vi "Material-Application-Constants.vi"() -> ()   [LabVIEW 2013]
panel:
  in  "Plugin Filename Pattern":string="Plugin-???-*.vi"
  in  "License Server Sandbox Request URI":string="https://apps.wirebirdlabs.com/license/deploy/sandbox"
  in  "License Server Registration URI":string="https://apps.wirebirdlabs.com/license/deploy/register"
  in  "Deploy Update Service Manifest URI":string="http://deploy.wirebirdlabs.com/OfficialReleases.manifest"
  out "Color.BG.Normal":u32(colorbox)=16777215
  out "Color.Selection":u32(colorbox)=16777224
  out "Color.BG.Fail":u32(colorbox)=16763594
  out "Color.BG.Success":u32(colorbox)=15204311
  out "Color.Text.Normal":u32(colorbox)=4276545
  out "Color.Text.Fail":u32(colorbox)=12517376
  out "Color.Text.Success":u32(colorbox)=3176192
  # "Colors"
  # "Endpoints"
  # "Plugin Constants"
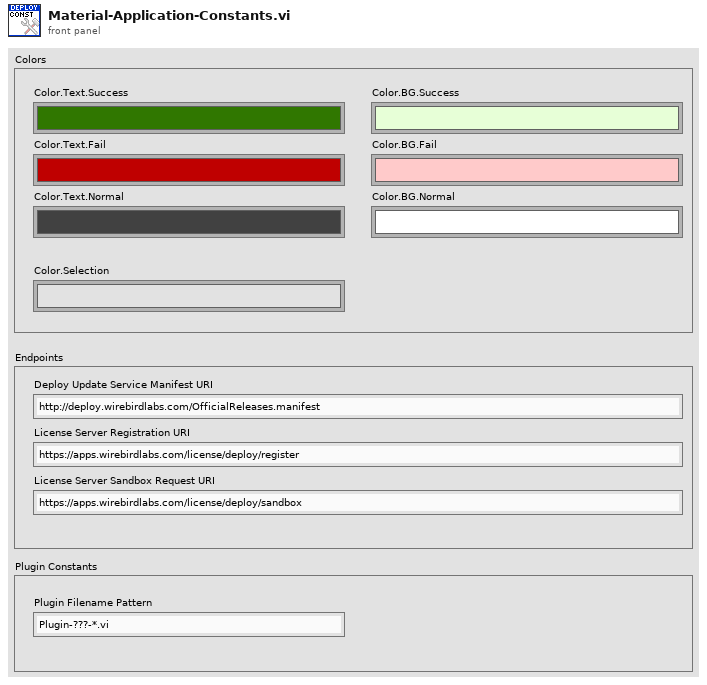
[diagram p1: front panel]
diagram:
